vi "ImportScan.vi"(8 "error in (no error)":errorcluster, 10 "Tuple":T1={"mouse_id"=1217.0, "exp_date"="2013-05-16", "scan_idx"=33.0, "file_name"="test", "scan_prog"="Imager", "aim"="other", "stim_engine"="None", "Lens"=0.0, "mag"=0.0, "laser_wavelength"=0.0, "attenuator_setting"=0.0, "x"=0.0, "y"=0.0, "z"=0.0, "surfz"=0.0, "scan_rotation"=0.0, "notes"="", "cell_patch"=0.0, "state"="", "problem_type"=""}, 11 "Database in":refnum<class "Database.lvclass">) -> (0 "error out":errorcluster, 3 "Database out":refnum<class "Database.lvclass">)   [LabVIEW 2012, in "Database.lvclass"]
uses:
  Database.lvclass
  Database.lvclass/Database.ctl
  <vilib>/addons/database/NI_Database_API.lvlib
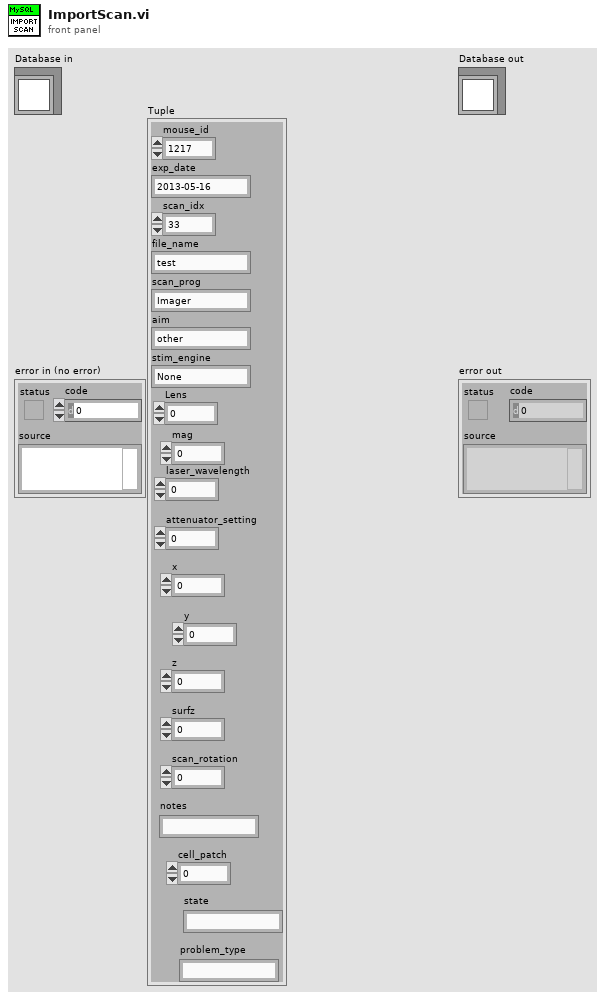
[diagram p1: front panel]
types:
  T1 = cluster{"mouse_id":dbl, "exp_date":string, "scan_idx":dbl, "file_name":string, "scan_prog":string, "aim":string, "stim_engine":string, "Lens":dbl, "mag":dbl, "laser_wavelength":dbl, "attenuator_setting":dbl, "x":dbl, "y":dbl, "z":dbl, "surfz":dbl, "scan_rotation":dbl, "notes":string, "cell_patch":dbl, "state":string, "problem_type":string}
  T2 = typedef "NI_Database_API.lvlib/Conn ObjectReference.ctl" = refnum<k1>
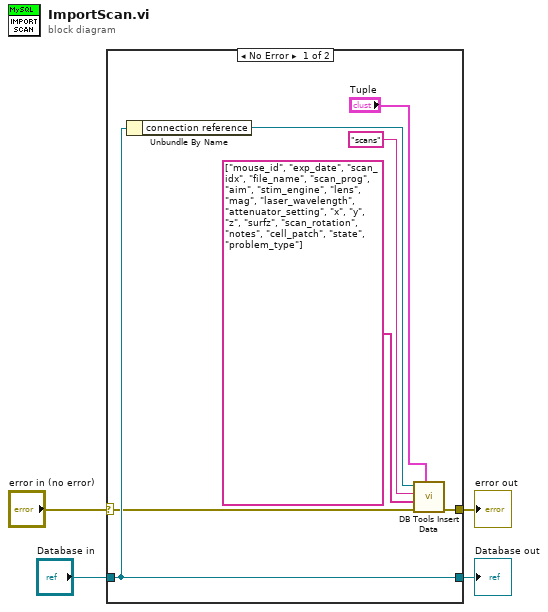
[diagram p0: block diagram]
diagram:
  n1 = case shown="No Error" "error in (no error)" {
    selector: "error in (no error)" -> [w8 w13]
    tunnel: [w7 w13] -> w3
    tunnel: [w11 w12] -> w1
    tunnel: "Database in" -> [w11 w12]
    frame No Error {
      n2 = Unbundle By Name(w11) -> ("connection reference"=w9:T2)
      n3 = call <vilib>:"DB Tools Insert Data.vi"("data"="Tuple", "error in (no error)"=w8, "columns"=string[] ["mouse_id", "exp_date", "scan_idx", "file_name", "scan_prog", "aim", "stim_engine", "lens", "mag", "laser_wavelength", "attenuator_setting", "x", "y", "z", "surfz", "scan_rotation", "notes", "cell_patch", "state", "problem_type"], "table"="scans", "connection reference"=w9) -> ("error out"=w7:errorcluster)  [unwired: 5 in, 1 out]
    }
    frame Error {
    }
  }
  "error out" <- w3
  "Database out" <- w1
